vi "FTW-JSON-Container-Traverse.vi"(0 "Container":refnum<class "FTW-Container.lvclass">, 1 "Options":T1={"Include Name"=FALSE, "Indent"=0, "Spaces"=4, "Pretty Print"=FALSE}, 7 "Name":string, 11 "error in":errorcluster) -> (4 "JSON String":string, 15 "error out":errorcluster)   [LabVIEW 2015]
uses:
  container/FTW-Container.lvclass
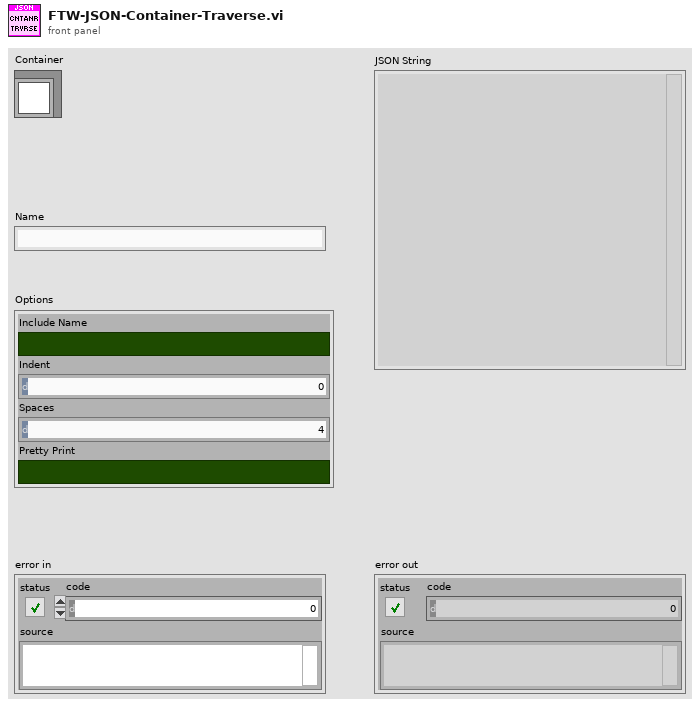
[diagram p1: front panel]
types:
  T1 = cluster{"Include Name":bool, "Indent":i32, "Spaces":i32, "Pretty Print":bool}
  T2 = typedef "FTW-Container.lvclass/FTW-Container-Type.ctl" = enum8{"invalid", "String", "Integer", "Real", "Object", "Array", "Boolean", "null"}
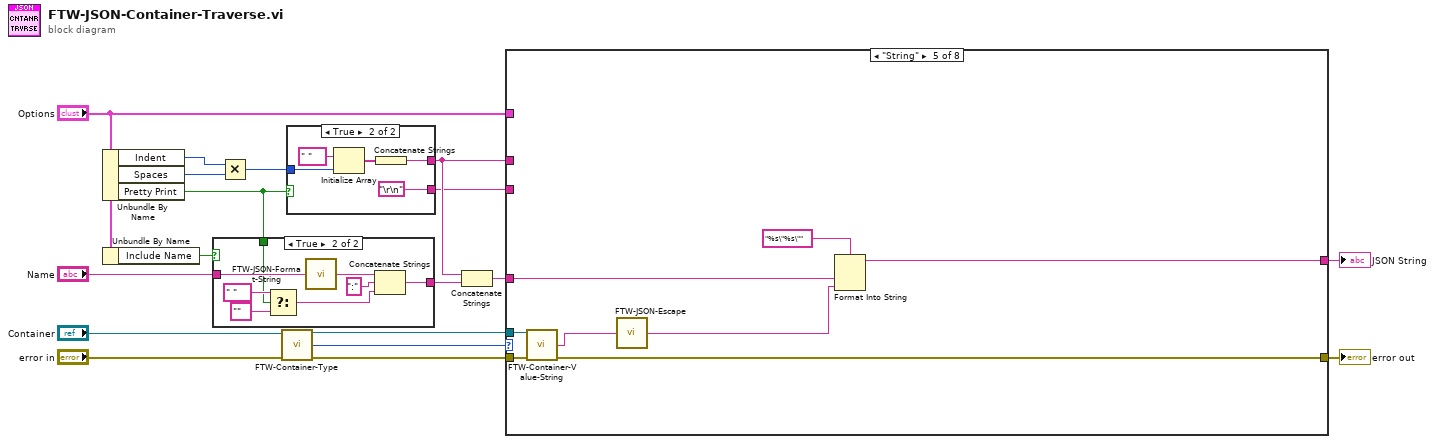
[diagram p0: block diagram]
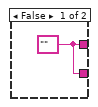
[diagram p2: hidden frame]
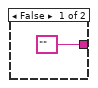
[diagram p3: hidden frame]
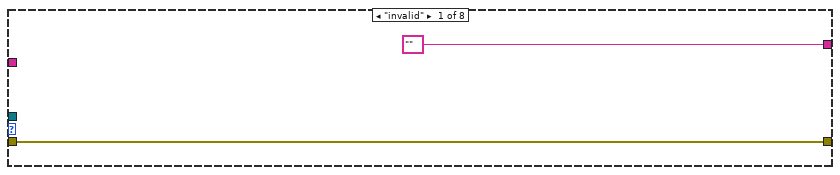
[diagram p4: hidden frame]
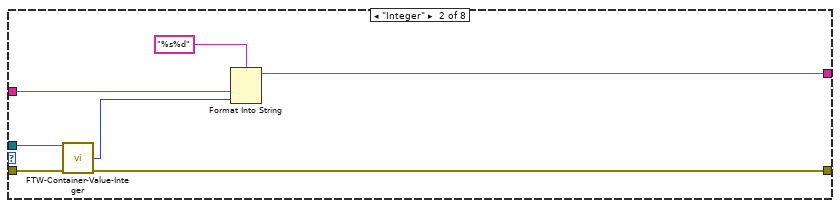
[diagram p5: hidden frame]
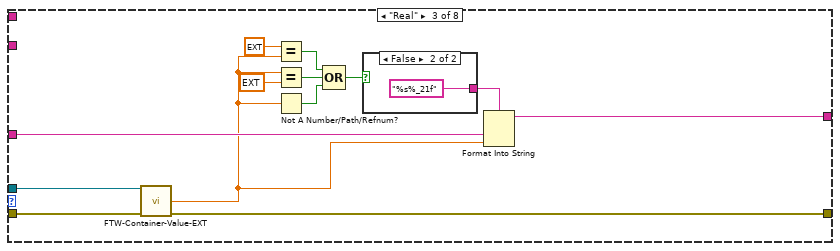
[diagram p6: hidden frame]
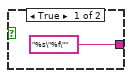
[diagram p7: hidden frame]
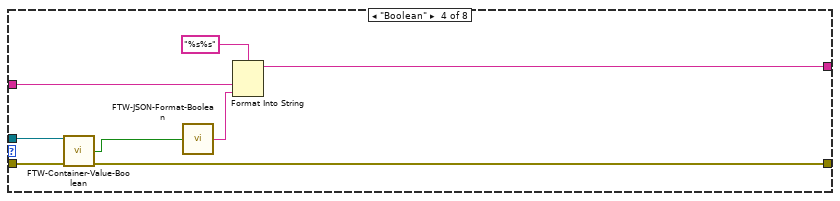
[diagram p8: hidden frame]
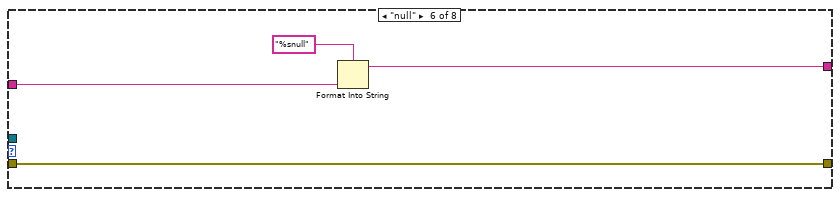
[diagram p9: hidden frame]
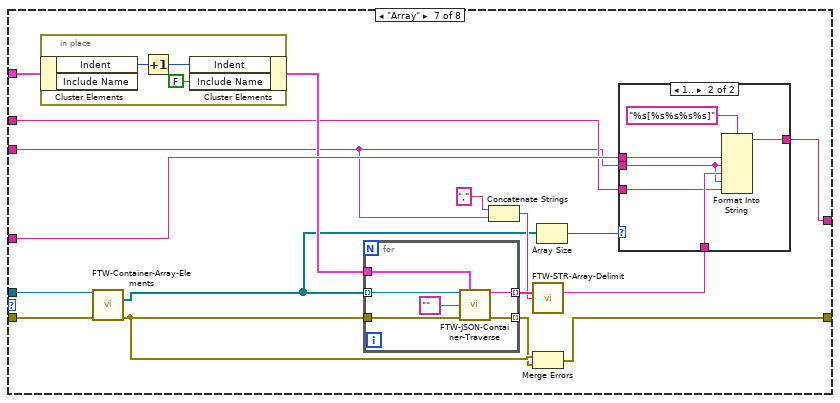
[diagram p10: hidden frame]
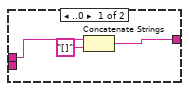
[diagram p11: hidden frame]
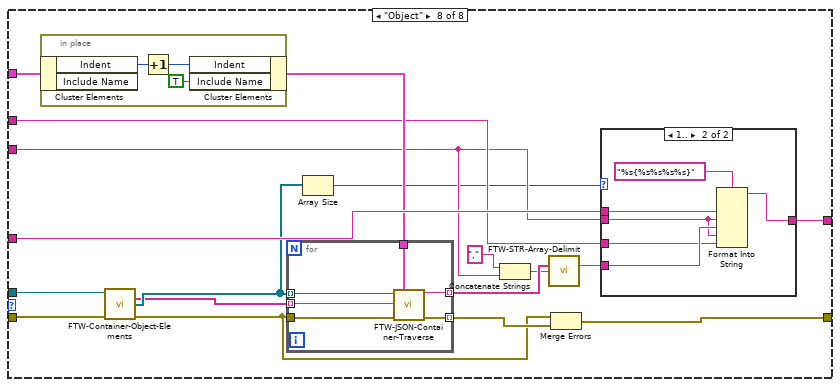
[diagram p12: hidden frame]
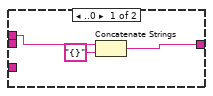
[diagram p13: hidden frame]
diagram:
  n1 = Unbundle By Name("Options") -> ("Indent"=w10:i32, "Spaces"=w12:i32, "Pretty Print"=w5:bool)
  n2 = Unbundle By Name("Options") -> ("Include Name"=w8:bool)
  n3 = case shown="True" w8 {
    tunnel: "Name" -> [_ w24]
    tunnel: ["" ("empty string") w27] -> w15
    tunnel: w5 -> [_ w21]
    frame False {
    }
    frame True {
      n4 = Select(t=" " ("empty string"), s=w21, f="" ("empty string")) -> (s? t:f=w20:string)
      n5 = call "FTW-JSON-Format-String.vi"("LabVIEW String"=w24) -> ("JSON String"=w25:string)
      n6 = Concatenate Strings(w25, ":" ("string"), w20) -> (w27:string)
    }
  }
  n7 = Multiply(x=w10, y=w12) -> (x*y=w11:i32)
  n8 = call "FTW-Container-Type.vi"("FTW-Container In"="Container", "error in"="error in") -> ("FTW-Container Out"=w2:refnum<class "FTW-Container.lvclass">, "Type"=w1:T2, "error out"=w4:errorcluster)  [unwired: 11 in]
  n9 = case shown="True" w5 {
    tunnel: w11 -> [_ w33]
    tunnel: [w28 w31] -> w9
    tunnel: [w28 "\r\n"] -> w7
    frame False {
      w28 = "" ("empty string")
    }
    frame True {
      n10 = Initialize Array(" " ("empty string"), w33) -> (w32:string[])
      n11 = Concatenate Strings(w32) -> (w31:string)
    }
  }
  n12 = Concatenate Strings(w9, w15) -> (w14:string)
  n13 = case shown="\"String\"" w1 {
    tunnel: w14 -> [_ w39 w50 w61 w69 w74 w90 w125]
    tunnel: w4 -> [w35 w42 w55 w65 w73 w77 w93 w130]
    tunnel: [w35 w38 w54 w60 w72 w77 w94 w123] -> w17
    tunnel: ["" ("empty string") w40 w51 w63 w70 w75 w92 w124] -> w16
    tunnel: w2 -> [_ w37 w53 w59 w67 _ w83 w115]
    tunnel: "Options" -> [_ _ _ _ _ _ w89 w122]
    tunnel: w9 -> [_ _ _ _ _ _ w87 w119]
    tunnel: w7 -> [_ _ _ _ _ _ w86 w118]
    frame "invalid" {
    }
    frame "Integer" {
      n14 = call "FTW-Container-Value-Integer.vi"("JSON"=w37, "error in"=w42) -> ("Value"=w36:i64, "error out"=w38:errorcluster)  [unwired: 11 in, 1 out]
      n15 = Format Into String(format string="%s%d", w39, w36) -> (resulting string=w40:string)  [unwired: 2 in, 1 out]
    }
    frame "Real" {
      n16 = call "FTW-Container-Value-EXT.vi"("JSON"=w53, "error in"=w55) -> ("Value"=w43:ext, "error out"=w54:errorcluster)  [unwired: 11 in, 1 out]
      n17 = Equal?(x=ext inf, y=w43) -> (x = y?=w47:bool)
      n18 = Equal?(x=w43, y=ext -inf) -> (x = y?=w49:bool)
      n19 = Not A Number/Path/Refnum?(number/path/refnum=w43) -> (NaN/Path/Refnum?=w46:bool)
      n20 = Compound Arithmetic op=OR(w47, w49, w46) -> (w48:bool)
      n21 = case shown="False" w48 {
        tunnel: ["%s\"%f\"" ("format string") "%s%_21f" ("format string")] -> w52
        frame True {
        }
        frame False {
        }
      }
      n22 = Format Into String(format string=w52, w50, w43) -> (resulting string=w51:string)  [unwired: 2 in, 1 out]
    }
    frame "Boolean" {
      n23 = call "FTW-Container-Value-Boolean.vi"("FTW-Container In"=w59, "error in"=w65) -> ("Value"=w58:bool, "error out"=w60:errorcluster)  [unwired: 11 in, 1 out]
      n24 = call "FTW-JSON-Format-Boolean.vi"("LabVIEW Boolean"=w58) -> ("JSON Boolean"=w62:string)
      n25 = Format Into String(format string="%s%s", w61, w62) -> (resulting string=w63:string)  [unwired: 2 in, 1 out]
    }
    frame "String" {
      n26 = call "FTW-Container-Value-String.vi"("JSON"=w67, "error in"=w73) -> ("Value"=w66:string, "error out"=w72:errorcluster)  [unwired: 11 in, 1 out]
      n27 = call "FTW-JSON-Escape.vi"("String"=w66) -> ("Escaped UTF-8 String"=w68:string)
      n28 = Format Into String(format string="%s\"%s\"", w69, w68) -> (resulting string=w70:string)  [unwired: 2 in, 1 out]
    }
    frame "null" {
      n29 = Format Into String(format string="%snull", w74) -> (resulting string=w75:string)  [unwired: 2 in, 1 out]
    }
    frame "Array" {
      n30 = in-place {
        n31 = in-place-cluster #1(w89) -> ("Indent"=w112:i32)  [unwired: 1 out]
        n32 = Increment(x=w112) -> (x+1=w111:i32)
        n33 = in-place-cluster #1("Indent"=w111, "Include Name"=FALSE) -> (w88:T1)
      }
      n34 = call "FTW-Container-Array-Elements.vi"("FTW-Container In"=w83, "error in"=w93) -> ("Array Elements"=w78:refnum<class "FTW-Container.lvclass">[], "error out"=w84:errorcluster)  [unwired: 11 in, 1 out]
      n35 = for {
        tunnel: w78 -> [w96] mode=indexing
        tunnel: [w99] -> w81 mode=indexing
        tunnel: w84 -> [w98]
        tunnel: [w100] -> w82 mode=indexing
        tunnel: w88 -> [w97]
        n36 = call "FTW-JSON-Container-Traverse.vi"("Container"=w96, "Options"=w97, "Name"="" ("empty string"), "error in"=w98) -> ("JSON String"=w99:string, "error out"=w100:errorcluster)  [unwired: 10 in]
      }
      n37 = Concatenate Strings("," ("Delimiter"), w86) -> (w79:string)
      n38 = call "FTW-STR-Array-Delimit.vi"("Array of Strings"=w81, "Delimiter"=w79) -> ("Delimited String"=w91:string)  [unwired: 13 in]
      n39 = Merge Errors(w84, w82) -> (w94:errorcluster)
      n40 = Array Size(array=w78) -> (size(s)=w85:i32)
      n41 = case shown="1.." w85 {
        tunnel: [w102 w108] -> w92
        tunnel: w91 -> [_ w107]
        tunnel: w90 -> [w103 w106]
        tunnel: w87 -> [_ w105]
        tunnel: w86 -> [_ w104]
        frame ..0 {
          n42 = Concatenate Strings(w103, "[]" ("string")) -> (w102:string)
        }
        frame 1.. {
          n43 = Format Into String(format string="%s[%s%s%s%s]", w106, w104, w107, w104, w105) -> (resulting string=w108:string)  [unwired: 2 in, 1 out]
        }
      }
    }
    frame "Object" {
      n44 = in-place {
        n45 = in-place-cluster #2(w122) -> ("Indent"=w142:i32)  [unwired: 1 out]
        n46 = Increment(x=w142) -> (x+1=w141:i32)
        n47 = in-place-cluster #2("Indent"=w141, "Include Name"=TRUE) -> (w121:T1)
      }
      n48 = call "FTW-Container-Object-Elements.vi"("FTW-Container In"=w115, "error in"=w130) -> ("Names"=w113:string[], "Object Elements"=w114:refnum<class "FTW-Container.lvclass">[], "error out"=w116:errorcluster)  [unwired: 10 in, 1 out]
      n49 = for {
        tunnel: [w146] -> w128 mode=indexing
        tunnel: w116 -> [w148]
        tunnel: [w147] -> w129 mode=indexing
        tunnel: w121 -> [w145]
        tunnel: w114 -> [w144] mode=indexing
        tunnel: w113 -> [w143] mode=indexing
        n50 = call "FTW-JSON-Container-Traverse.vi"("Container"=w144, "Options"=w145, "Name"=w143, "error in"=w148) -> ("JSON String"=w146:string, "error out"=w147:errorcluster)  [unwired: 10 in]
      }
      n51 = Array Size(array=w114) -> (size(s)=w117:i32)
      n52 = Concatenate Strings("," ("Delimiter"), w118) -> (w120:string)
      n53 = call "FTW-STR-Array-Delimit.vi"("Array of Strings"=w128, "Delimiter"=w120) -> ("Delimited String"=w126:string)  [unwired: 13 in]
      n54 = Merge Errors(w116, w129) -> (w123:errorcluster)
      n55 = case shown="1.." w117 {
        tunnel: w126 -> [_ w139]
        tunnel: w125 -> [w133 w137]
        tunnel: [w132 w136] -> w124
        tunnel: w119 -> [_ w135]
        tunnel: w118 -> [_ w134]
        frame ..0 {
          n56 = Concatenate Strings(w133, "{}" ("string")) -> (w132:string)
        }
        frame 1.. {
          n57 = Format Into String(format string="%s{%s%s%s%s}", w137, w134, w139, w134, w135) -> (resulting string=w136:string)  [unwired: 2 in, 1 out]
        }
      }
    }
  }
  "error out" <- w17
  "JSON String" <- w16
